vi "convertMFCInputBytes.vi"(6 "FullScale":dbl=24576.0, 7 "SCCM":dbl=500.0, 8 "MFC Bytes":u8[](array[numeric])) -> (1 "Actuator Drive Valve":i16, 2 "Setpoint (SCCM)":dbl, 3 "Flow (SCCM)":dbl, 4 "Actuator Override":u8, 5 "Status":bool[](array[boolean]))   [LabVIEW 2011]
uses:
  <vilib>/imath/engines/lvmath2/RunTimeEngine/NodeEndStatement/NIMS_NodeEndStatement_Output.vi
  <instcachedir>/0/NIMS_NodeEndStatement_Output_53EC0D466D134D7ABD903AC30B43404B.lvgen/NIMS_NodeEndStatement_Output_53EC0D466D134D7ABD903AC30B43404B_001.vi
  <vilib>/imath/engines/lvmath2/RunTimeEngine/ErrorHandling/NIMS_Finalize Error.vi
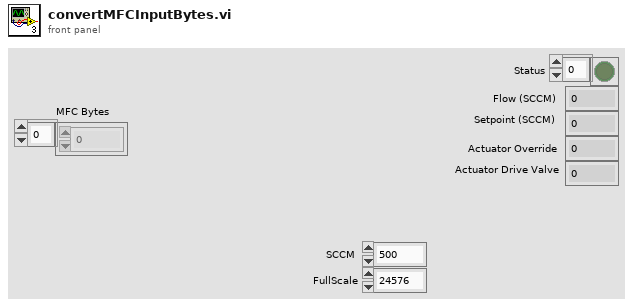
[diagram p1: front panel]
types:
  T1 = cluster{"[0]":u8, "[1]":u8, "[2]":u8, "[3]":u8, "[4]":u8, "[5]":u8, "[6]":u8, "[7]":u8}
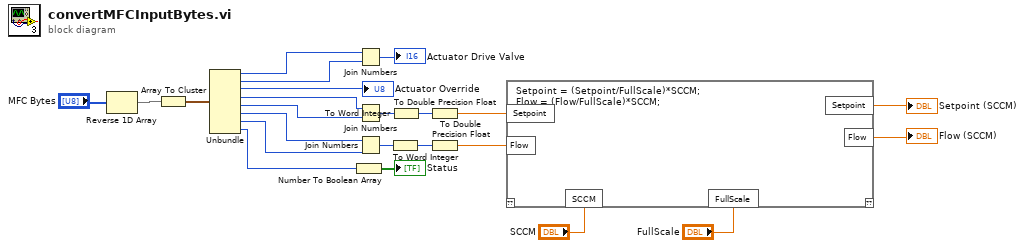
[diagram p0: block diagram]
diagram:
  n1 = Reverse 1D Array(array="MFC Bytes") -> (reversed array=w14:u8[])
  n2 = Array To Cluster(array=w14) -> (cluster=w15:T1)
  n3 = Unbundle(w15) -> ("[0]"=w5:u8, "[1]"=w6:u8, "[2]"=→"Actuator Override":u8, "[3]"=w8:u8, "[4]"=w9:u8, "[5]"=w10:u8, "[6]"=w11:u8, "[7]"=w12:u8)
  n4 = Number To Boolean Array(number=w12) -> (Boolean array=→"Status":bool[])
  n5 = Join Numbers(hi=w5, lo=w6) -> ((hi.lo)=→"Actuator Drive Valve":u16)
  n6 = Join Numbers(hi=w8, lo=w9) -> ((hi.lo)=w1:u16)
  n7 = Join Numbers(hi=w10, lo=w11) -> ((hi.lo)=w2:u16)
  n8 = To Word Integer(number=w2) -> (16bit integer=w3:i16)
  n9 = To Word Integer(number=w1) -> (16bit integer=w4:i16)
  n10 = To Double Precision Float(number=w4) -> (double precision float=w21:dbl)
  n11 = To Double Precision Float(number=w3) -> (double precision float=w20:dbl)
  n12 = mathscript code="Setpoint = (Setpoint/FullScale)*SCCM;\nFlow = (Flow/FullScale)*SCCM;"("Flow"=w20, "Setpoint"=w21, "SCCM"="SCCM", "FullScale"="FullScale") -> ("Flow"=→"Flow (SCCM)":dbl, "Setpoint"=→"Setpoint (SCCM)":dbl)  [unwired: 1 in, 1 out]
